vi "Render Variable.vi"(8 "Error In":errorcluster, 10 "Tag":refnum<class "Variable.lvclass">, 11 "Renderer In":refnum<class "Renderer.lvclass">) -> (0 "Error Out":errorcluster, 2 "Output":string, 3 "Renderer Out":refnum<class "Renderer.lvclass">)   [LabVIEW 2018, in "Toolkit.lvlib" / "Renderer.lvclass"]
uses:
  Renderer.lvclass
  Nodes/Variable/Variable.lvclass
  Nodes/Variable/Variable.lvclass/Variable.ctl
  Data/String/String.lvclass
  Data/String/String.lvclass/String.ctl
  Data/Datum/Datum.lvclass
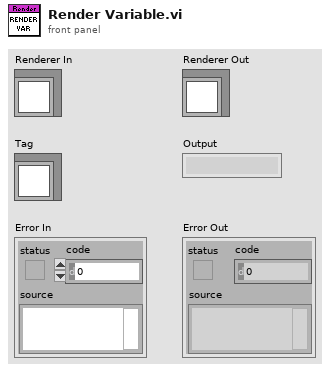
[diagram p1: front panel]
types:
  T1 = typedef "Toolkit.lvlib/Data.lvlib/Types.ctl" = enum16{"Array", "Boolean", "Function", "Map", "Null", "Pair", "Path", "String", "Unknown"}
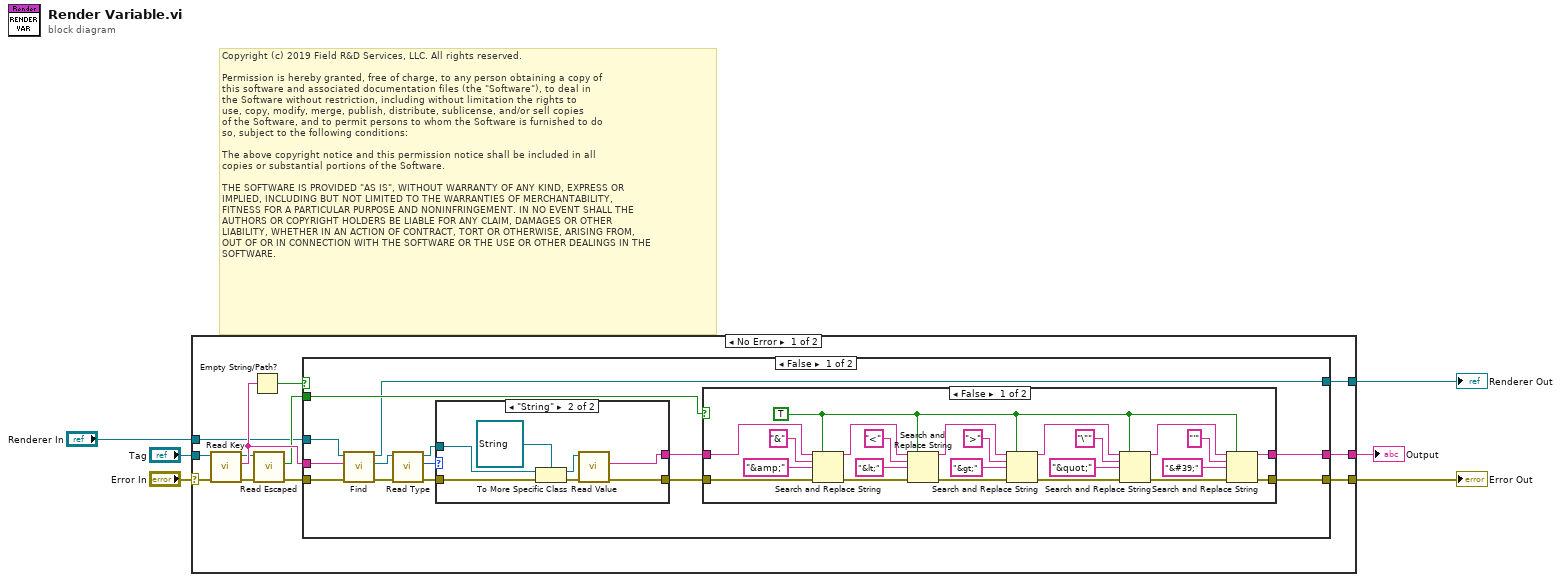
[diagram p0: block diagram]
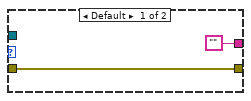
[diagram p2: hidden frame]
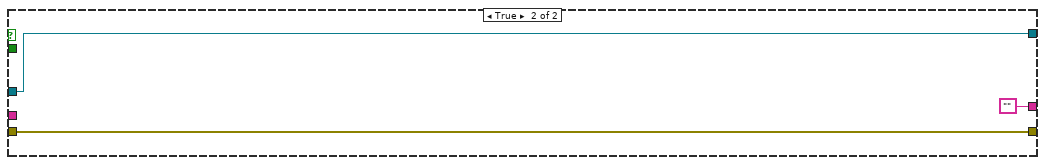
[diagram p4: hidden frame]
diagram:
  # "Copyright (c) 2019 Field R&D Services, LLC. All rights reserved.\n\nPermission is hereby granted, free of charge, to any person obtaining a copy of\nthis software and associated documentation files (the \"Software\"), to deal in\nthe Software without restriction, including without limitation the rights to\nuse, copy, modify, merge, publish, distribute, sublicense, and/or sell copies\nof the Software, and to permit persons to whom the Software is furnished to do\nso, subject to the following conditions:\n\nThe above copyright notice and this permission notice shall be included in all\ncopies or substantial portions of the Software.\n\nTHE SOFTWARE IS PROVIDED \"AS IS\", WITHOUT WARRANTY OF ANY KIND, EXPRESS OR\nIMPLIED, INCLUDING BUT NOT LIMITED TO THE WARRANTIES OF MERCHANTABILITY,\nFITNESS FOR A PARTICULAR PURPOSE AND NONINFRINGEMENT. IN NO EVENT SHALL THE\nAUTHORS OR COPYRIGHT HOLDERS BE LIABLE FOR ANY CLAIM, DAMAGES OR OTHER\nLIABILITY, WHETHER IN AN ACTION OF CONTRACT, TORT OR OTHERWISE, ARISING FROM,\nOUT OF OR IN CONNECTION WITH THE SOFTWARE OR THE USE OR OTHER DEALINGS IN THE\nSOFTWARE."
  n1 = case shown="No Error" "Error In" {
    selector: "Error In" -> [w10 w71]
    tunnel: "Tag" -> [w11 _]
    tunnel: [w7 w71] -> w4
    tunnel: "Renderer In" -> [w12 w70]
    tunnel: [w9 w70] -> w1
    tunnel: [w8 _] -> w2
    frame No Error {
      n2 = call "Read Key.vi"("Error In"=w10, "Variable In"=w11) -> ("Error Out"=w15:errorcluster, "Key"=w17:string, "Variable Out"=w16:refnum<class "Variable.lvclass">)  [unwired: 7 in]
      n3 = Empty String/Path?(string/path=w17) -> (empty?=w18:bool)
      n4 = call "Read Escaped.vi"("Error In"=w15, "Variable In"=w16) -> ("Error Out"=w13:errorcluster, "Escaped"=w14:bool)  [unwired: 7 in, 1 out]
      n5 = case shown="False" w18 {
        tunnel: [w32 w69] -> w7
        tunnel: [w31 ""] -> w8
        tunnel: w14 -> [w30 _]
        tunnel: w17 -> [w27 _]
        tunnel: w13 -> [w26 w69]
        tunnel: [w24 w67] -> w9
        tunnel: w12 -> [w19 w67]
        frame False {
          n6 = call "Find.vi"("Error In"=w26, "Key"=w27, "Renderer In"=w19) -> ("Error Out"=w22:errorcluster, "Datum"=w25:refnum<class "Datum.lvclass">, "Renderer Out"=w24:refnum<class "Renderer.lvclass">)  [unwired: 5 in, 1 out]
          n7 = call-dynamic "Read Type.vi"("Error In"=w22, "Datum In"=w25) -> ("Error Out"=w20:errorcluster, "Type"=w21:T1, "Datum Out"=w23:refnum<class "Datum.lvclass">)  [unwired: 7 in]
          n8 = case shown="\"String\"" w21 {
            tunnel: w20 -> [w34 w41]
            tunnel: w23 -> [_ w39]
            tunnel: [w34 w36] -> w29
            tunnel: ["" w35] -> w28
            frame Default {
            }
            frame "String" {
              n9 = To More Specific Class(target class=refnum<class "String.lvclass"> refnum ("Toolkit.lvlib:Data.lvlib:String.lvclass"), reference=w39, error in=w41) -> (specific class reference=w37:refnum<class "String.lvclass">, error out=w38:errorcluster)
              n10 = call "Read Value.vi"("Error In"=w38, "String In"=w37) -> ("Error Out"=w36:errorcluster, "Value"=w35:string)  [unwired: 7 in, 1 out]
            }
          }
          n11 = case shown="False" w30 {
            tunnel: [w45 w65] -> w32
            tunnel: [w44 w66] -> w31
            tunnel: w29 -> [w43 w65]
            tunnel: w28 -> [w42 w66]
            frame False {
              w48 = TRUE ("replace all? (F)")
              n12 = Search and Replace String(replace all?=w48, input string=w42, search string="&", replace string="&amp;" ("replace string (\"\")"), error in=w43) -> (result string=w60:string, error out=w59:errorcluster)  [unwired: 3 in, 2 out]
              n13 = Search and Replace String(replace all?=w48, input string=w60, search string="<", replace string="&lt;" ("replace string (\"\")"), error in=w59) -> (result string=w57:string, error out=w58:errorcluster)  [unwired: 3 in, 2 out]
              n14 = Search and Replace String(replace all?=w48, input string=w57, search string=">", replace string="&gt;" ("replace string (\"\")"), error in=w58) -> (result string=w53:string, error out=w54:errorcluster)  [unwired: 3 in, 2 out]
              n15 = Search and Replace String(replace all?=w48, input string=w53, search string="\"" ("replace string (\"\")"), replace string="&quot;" ("replace string (\"\")"), error in=w54) -> (result string=w50:string, error out=w49:errorcluster)  [unwired: 3 in, 2 out]
              n16 = Search and Replace String(replace all?=w48, input string=w50, search string="'", replace string="&#39;" ("replace string (\"\")"), error in=w49) -> (result string=w44:string, error out=w45:errorcluster)  [unwired: 3 in, 2 out]
            }
            frame True {
            }
          }
        }
        frame True {
        }
      }
    }
    frame Error {
    }
  }
  "Error Out" <- w4
  "Output" <- w2
  "Renderer Out" <- w1
